vi "Create Tables.vi"(8 "error in (no error)":errorcluster, 11 "Config-Sqlite in":refnum<class "Config-Sqlite.lvclass">) -> (0 "error out":errorcluster, 3 "Config-Sqlite out":refnum<class "Config-Sqlite.lvclass">)   [LabVIEW 2020, in "CDM-Config.lvlib" / "Config-Sqlite.lvclass"]
uses:
  Config-Sqlite.lvclass
  <vilib>/drjdpowell/SQLite Library/SQLite.lvlib
  <vilib>/drjdpowell/SQLite Library/SQL Connection/Execute SQL (No results).vi
  <vilib>/drjdpowell/SQLite Library/SQL Connection/Connection.lvclass
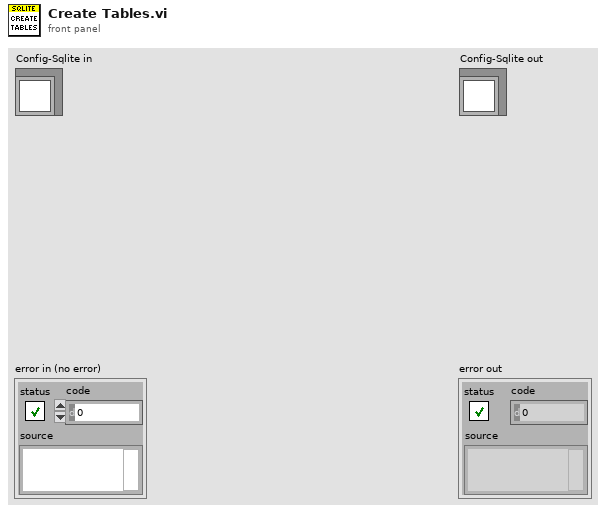
[diagram p1: front panel]
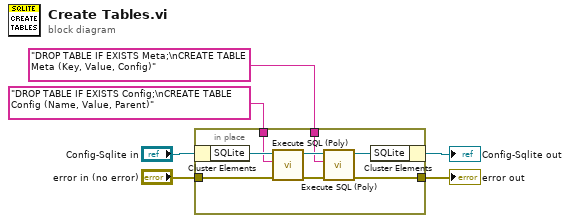
[diagram p0: block diagram]
diagram:
  n1 = in-place {
    in-place-border: "DROP TABLE IF EXISTS Config;\nCREATE TABLE Config (Name, Value, Parent)" -> [w7]
    in-place-border: "error in (no error)" -> [w14]
    in-place-border: "DROP TABLE IF EXISTS Meta;\nCREATE TABLE Meta (Key, Value, Config)" -> [w11]
    in-place-border: [w10] -> w3
    n2 = in-place-cluster #1("Config-Sqlite in") -> ("SQLite"=w9:refnum<class "Connection.lvclass">)
    n3 = call-poly <vilib>:"Execute SQL (Poly).vi"("error in (no error)"=w14, "SQL"=w7, "SQLite Connection in"=w9) -> ("error out"=w12:errorcluster, "SQLite Connection"=w13:refnum<class "Connection.lvclass">)  [unwired: 7 in]
    n4 = call-poly <vilib>:"Execute SQL (Poly).vi"("error in (no error)"=w12, "SQL"=w11, "SQLite Connection in"=w13) -> ("error out"=w10:errorcluster, "SQLite Connection"=w8:refnum<class "Connection.lvclass">)  [unwired: 7 in]
    n5 = in-place-cluster #1("SQLite"=w8) -> (→"Config-Sqlite out":refnum<class "Config-Sqlite.lvclass">)
  }
  "error out" <- w3
